vi "NI VeriStand - Send Workspace Tool Message (Byte Array).vi"(6 "Timeout ms (10000)":u32=10000, 7 "Workspace Tool Path":path, 8 "error in (no error)":errorcluster, 9 "Data":u8[](array[numeric]), 10 "Command":string, 11 "Project Ref in":T1) -> (0 "error out":errorcluster, 1 "Response":u8[](array[numeric]), 3 "Project Ref out":T1)   [LabVIEW 2020, in "NI_VS Project ExecutionAPI.lvlib"]
doc: "Sends a message or command to a Workspace tool for an NI VeriStand project, as well as data required by the case that handles the command. You can use this method with any Workspace tool that registers to receive the command you specify."
uses:
  <vilib>/NI VeriStand/Execution/Project/NI_VS Project ExecutionAPI.lvlib
  <vilib>/NI VeriStand/Execution/Project/Project Ref.ctl
  NationalInstruments.VeriStand.ClientAPI
  NationalInstruments.VeriStand
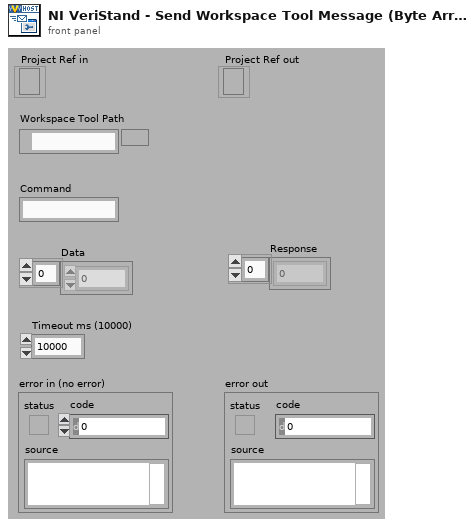
[diagram p1: front panel]
types:
  T1 = typedef "NI_VS Project ExecutionAPI.lvlib/Project Ref.ctl" = refnum<k24>
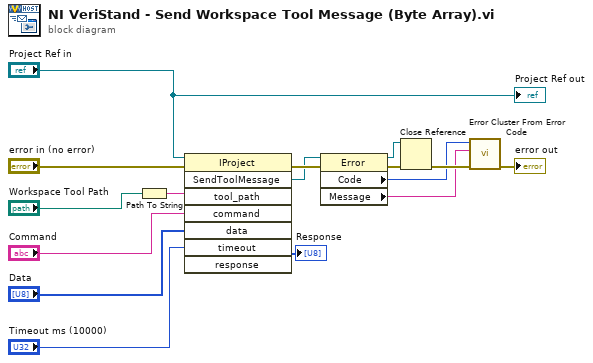
[diagram p0: block diagram]
diagram:
  n1 = Path To String(path="Workspace Tool Path") -> (string=w5:string)
  n2 = invoke class="IProject" method="SendToolMessage"(reference="Project Ref in", error in="error in (no error)", "tool_path"=w5, "command"="Command", "data"="Data", "timeout"="Timeout ms (10000)") -> (error out=w14:errorcluster, "SendToolMessage"=w9:refnum<k24>, "response"=→"Response":u8[])  [unwired: 2 in, 5 out]
  n3 = property class="Error"(reference=w9, error in=w14) -> (reference out=w12:refnum<k24>, error out=w13:errorcluster, "Code"=w8:u32, "Message"=w7:string)
  n4 = Close Reference(reference=w12, error in (no error)=w13) -> (error out=w11:errorcluster)
  n5 = call <vilib>:"Error Cluster From Error Code.vi"("error in (no error)"=w11, "error message (\"\")"=w7, "error code (0)"=w8) -> ("error out"=→"error out":errorcluster)  [unwired: 6 in]
  "Project Ref out" <- "Project Ref in"
